vi "Method Dialog_Setup Show Options.vi"(6 "Properties for Tree In":T1(array[cluster])=[{"Label"="a", "Tag"="a", "Property Type"=enum."Base", "Indent"=0, "Can Read?"=TRUE, "Can Write?"=TRUE, "Is Read?"=FALSE, "Is Write?"=TRUE, "Inactive Parent?"=FALSE, "Unwired?"=FALSE}, {"Label"="b", "Tag"="b", "Property Type"=enum."Scripting", "Indent"=0, "Can Read?"=TRUE, "Can Write?"=FALSE, "Is Read?"=FALSE, "Is Write?"=FALSE, "Inactive Parent?"=FALSE, "Unwired?"=FALSE}, {"Label"="c", "Tag"="c", "Property Type"=enum."Base", "Indent"=0, "Can Read?"=TRUE, "Can Write?"=TRUE, "Is Read?"=FALSE, "Is Write?"=FALSE, "Inactive Parent?"=FALSE, "Unwired?"=FALSE}, {"Label"="d", "Tag"="d", "Property Type"=enum."Private", "Indent"=0, "Can Read?"=TRUE, "Can Write?"=FALSE, "Is Read?"=FALSE, "Is Write?"=FALSE, "Inactive Parent?"=FALSE, "Unwired?"=FALSE}, {"Label"="E", "Tag"="E", "Property Type"=enum."Base", "Indent"=0, "Can Read?"=TRUE, "Can Write?"=TRUE, "Is Read?"=FALSE, "Is Write?"=TRUE, "Inactive Parent?"=FALSE, "Unwired?"=FALSE}, {"Label"="f", "Tag"="f", "Property Type"=enum."Base", "Indent"=0, "Can Read?"=TRUE, "Can Write?"=FALSE, "Is Read?"=FALSE, "Is Write?"=FALSE, "Inactive Parent?"=FALSE, "Unwired?"=FALSE}], 8 "error in (no error)":errorcluster, 11 "Cluster in":refnum<vi>) -> (0 "error out":errorcluster)   [LabVIEW 2023]
doc: "Show/hide option booleans for \n\n--Show script/schow private\n--Select unwired termainls (remove items action)"
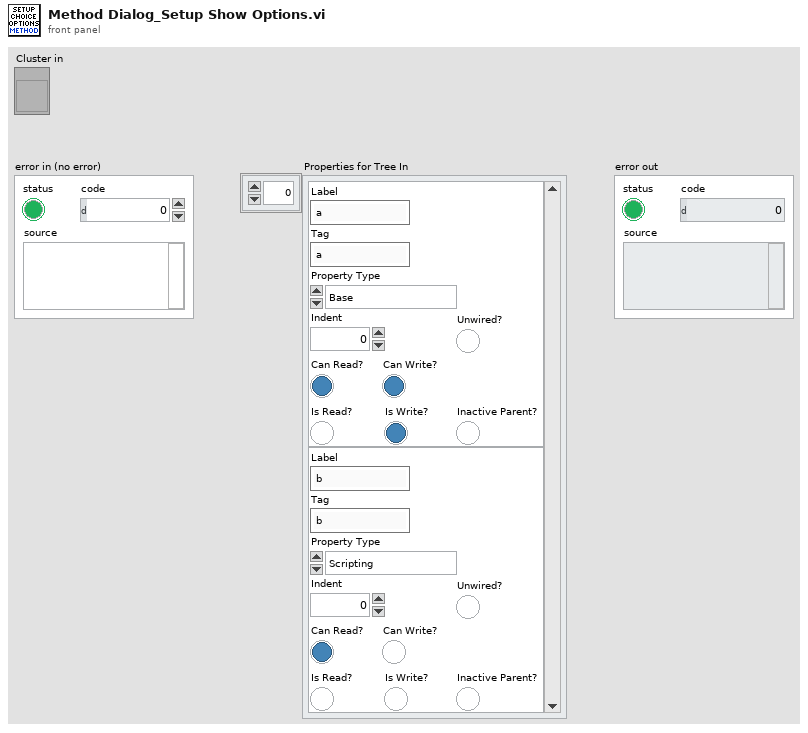
[diagram p1: front panel]
types:
  T1 = cluster{"Label":string, "Tag":string, "Property Type":enum16{"Unknown", "Base", "Scripting", "Private", "Deprecated", "None", "Divider"}, "Indent":u16, "Can Read?":bool, "Can Write?":bool, "Is Read?":bool, "Is Write?":bool, "Inactive Parent?":bool, "Unwired?":bool}[]
  T2 = enum8{"Enabled", "Disabled", "Disabled and Grayed Out"}
  T3 = enum16{"Unknown", "Base", "Scripting", "Private", "Deprecated", "None", "Divider"}
  T4 = cluster{"Show Scripting":bool, "Show Private":bool}
  T5 = enum8{"Enabled", "Disabled", "Disabled and Grayed Out"}[]
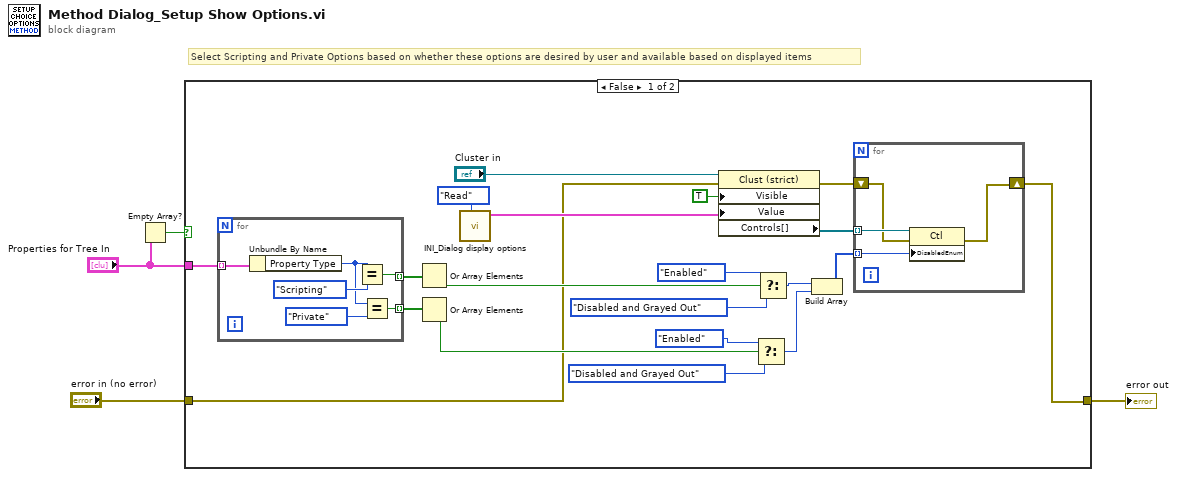
[diagram p0: block diagram]
diagram:
  # "Select Scripting and Private Options based on whether these options are desired by user and available based on displayed items"
  n1 = Empty Array?(array="Properties for Tree In") -> (empty?=w4:bool)
  n2 = case shown="False" w4 {
    tunnel: "Properties for Tree In" -> [w23 _]
    tunnel: "error in (no error)" -> [w7 w35]
    tunnel: [w5 w35] -> w1
    frame False {
      n3 = for {
        tunnel: w23 -> [w34] mode=indexing
        tunnel: [w32] -> w22 mode=indexing
        tunnel: [w29] -> w21 mode=indexing
        n4 = Unbundle By Name(w34) -> ("Property Type"=w31:T3)
        n5 = Equal?(x=w31, y=T3."Scripting" ("Property Type")) -> (x = y?=w32:bool)
        n6 = Equal?(x=w31, y=T3."Private" ("Property Type")) -> (x = y?=w29:bool)
      }
      n7 = Or Array Elements(Boolean array=w22) -> (logical OR=w20:bool)
      n8 = Or Array Elements(Boolean array=w21) -> (logical OR=w19:bool)
      n9 = call "INI_Dialog display options.vi"("File Action"=enum16{"Read", "Write"}."Read") -> ("Display Options Out"=w18:T4)  [unwired: 10 in]
      n10 = property class="Clust (strict)"(reference="Cluster in", error in=w7, "Visible"=TRUE, "Value"=w18) -> (error out=w6:errorcluster, "Controls[]"=w15:refnum<vi>[])  [unwired: 1 out]
      n11 = Select(t=T2."Enabled" ("Disabled"), s=w19, f=T2."Disabled and Grayed Out" ("Disabled")) -> (s? t:f=w10:T2)
      n12 = Select(t=T2."Enabled" ("Disabled"), s=w20, f=T2."Disabled and Grayed Out" ("Disabled")) -> (s? t:f=w11:T2)
      n13 = Build Array(w11, w10) -> (w8:T5)
      n14 = for {
        tunnel: w15 -> [w28] mode=indexing
        tunnel: w8 -> [w27] mode=indexing
        shift-right: [w25] -> w5
        shift-left: w6 -> [w26]
        n15 = property class="Ctl"(reference=w28, error in=w26, "DisabledEnum"=w27) -> (error out=w25:errorcluster)  [unwired: 1 out]
      }
    }
    frame True {
    }
  }
  "error out" <- w1
